vi "data_save.vi"() -> ()   [LabVIEW 2014]
panel:
  out "波形图表":waveform(dbl)[](graph)
  out "输出信号特征参数":dbl[](array[numeric])
  in  "Path":path
  in  "布尔":bool
  in  "路径":path
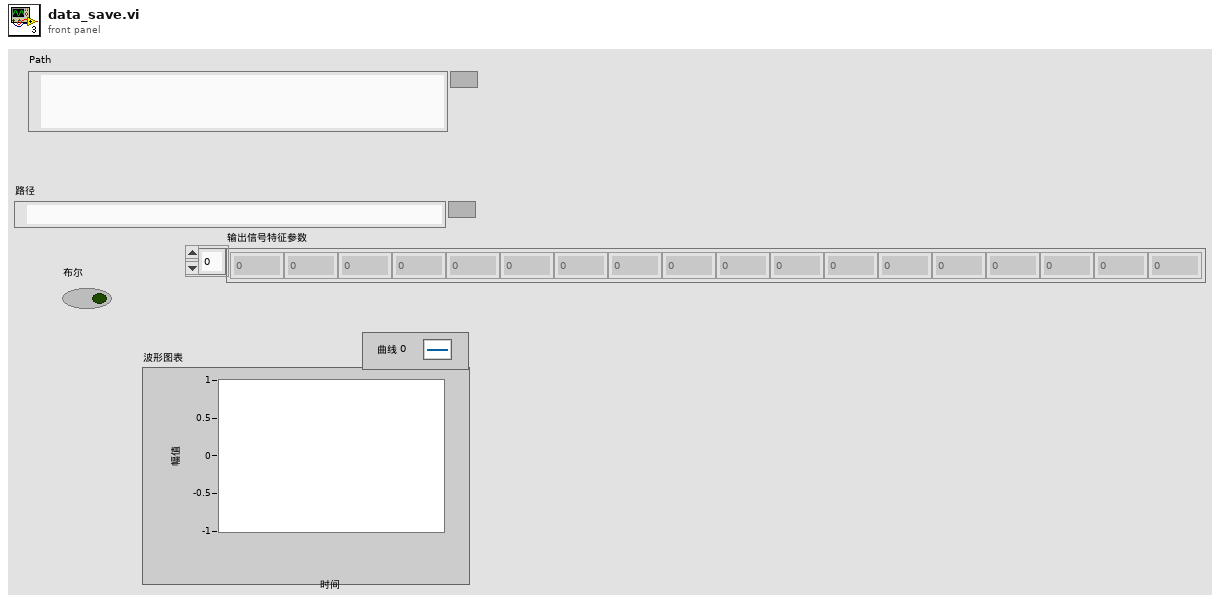
[diagram p1: front panel]
types:
  T1 = enum16{"open", "replace", "create", "open or create", "replace or create", "replace or create with confirmation"}
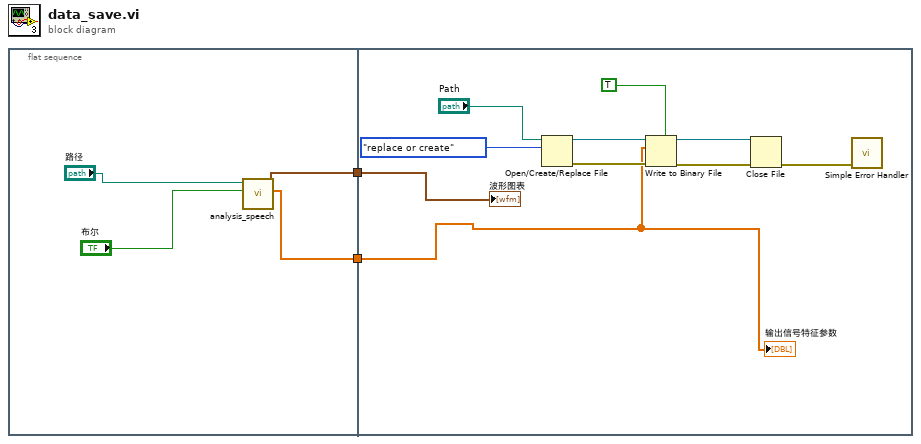
[diagram p0: block diagram]
diagram:
  n1 = flat-sequence {
    tunnel: [w4] -> w2
    tunnel: [w3] -> w1
    tunnel: w2 -> [w8]
    tunnel: w1 -> [w7]
    frame #0 {
      n2 = call "analysis_speech.vi"("布尔"="布尔", "文件路径（使用对话框）"="路径") -> ("数组"=w4:dbl[], "波形图表"=w3:waveform(dbl)[])  [unwired: 8 in]
    }
    frame #1 {
      n3 = Open/Create/Replace File(file path (use dialog)="Path", operation (0:open)=T1."replace or create") -> (refnum out=w14:refnum<file>, error out=w11:errorcluster)  [unwired: 4 in, 1 out]
      n4 = Write to Binary File(file (use dialog)=w14, data=w8, error in=w11, 5:TRUE ("prepend array or string size? (T)")) -> (refnum out=w15:refnum<file>, error out=w10:errorcluster)  [unwired: 2 in, 1 out]
      n5 = Close File(refnum=w15, error in=w10) -> (error out=w9:errorcluster)  [unwired: 1 out]
      n6 = call <vilib>:"Simple Error Handler.vi"("error in (no error)"=w9) -> ()  [unwired: 4 in, 5 out]
      "输出信号特征参数" <- w8
      "波形图表" <- w7
    }
  }
